vi "Lab Panel V5.28.vi"() -> ()   [LabVIEW 2013] (continued)
                            n1774 = local write "run lab05-2"(w3318) -> ()
                            n1775 = local write "DISP LAB05-2"(w3321) -> ()
                          }
                          frame #1 {
                            n1776 = TDMS Close(11:w3322) -> (0:w3323:errorcluster)  [unwired: 1 in, 1 out]
                            n1777 = local write "data file error"(w3323) -> ()
                          }
                          frame #2 {
                            n1778 = stacked-sequence {
                              tunnel: "LAB05-2" -> [w3331 w3337]
                              tunnel: w3328 -> [_ w3336]
                              tunnel: w3327 -> [_ w3335]
                              tunnel: w3326 -> [_ w3334]
                              tunnel: w3325 -> [_ w3333]
                              tunnel: w3324 -> [_ w3332]
                              frame #0 {
                                n1779 = call "sub vi - defrag tdms v1.vi"("panel id"=w3331) -> ("error out"=w3330:errorcluster)  [unwired: 10 in]
                                n1780 = local write "data file error"(w3330) -> ()
                              }
                              frame #1 {
                                n1781 = Bundle("STATUS"=w3336, "OUT SERVER ADDRESS"=w3335, "FROM ACCOUNT"=w3334, "Mail Test File To:"=w3333, "Mail Test Fail"=w3332) -> (w3339:T26)  [unwired: 1 in]
                                n1782 = call "Save data file (pass-fail) v5.vi"("Input Cluster"=w3339, "panel id"=w3337) -> ("network file save error"=w3338:errorcluster)  [unwired: 8 in, 1 out]
                                n1783 = local write "data file error"(w3338) -> ()
                              }
                            }
                          }
                        }
                      }
                    }
                  }
                }
              }
            }
            n1784 = global write "Global display 2.vi" "Mail test file to:"(w2847) -> ()
            n1785 = local read "Network Directory"() -> (w2853:path)
            n1786 = global write "Global 1.vi" "Network Drive"(w2853) -> ()
          }
          frame #8 {
            # "disable functions"
            n1787 = stacked-sequence {
              tunnel: w3349 -> [w3363 _ w3420]
              tunnel: w3348 -> [w3358 _ w3419]
              tunnel: w3347 -> [w3357 _ w3418]
              tunnel: w3346 -> [w3355 _ w3417]
              tunnel: w3345 -> [w3356 _ w3416]
              tunnel: w3344 -> [_ w3380 w3415]
              tunnel: w3343 -> [_ w3381 w3414]
              tunnel: w3342 -> [_ w3382 w3413]
              tunnel: w3341 -> [_ w3383 w3412]
              tunnel: w3340 -> [_ w3384 w3411]
              frame #0 {
                n1788 = Select(t=2, s=w3355, f=0) -> (s? t:f=w3351:i32)
                n1789 = Select(t=2, s=w3357, f=0) -> (s? t:f=w3352:i32)
                n1790 = Select(t=2, s=w3356, f=0) -> (s? t:f=w3350:i32)
                n1791 = Select(t=2, s=w3363, f=0) -> (s? t:f=w3354:i32)
                n1792 = Select(t=2, s=w3358, f=0) -> (s? t:f=w3353:i32)
                n1793 = property on="SELECT LAB02-2" class="RadioBtnsControl (strict)"("DisabledEnum"=w3351) -> ()  [unwired: 2 in, 2 out]
                n1794 = property on="SELECT LAB02-1" class="RadioBtnsControl (strict)"("DisabledEnum"=w3352) -> ()  [unwired: 2 in, 2 out]
                n1795 = property on="SELECT LAB03-1" class="RadioBtnsControl (strict)"("DisabledEnum"=w3350) -> ()  [unwired: 2 in, 2 out]
                n1796 = property on="SELECT LAB01-1" class="RadioBtnsControl (strict)"("DisabledEnum"=w3354) -> ()  [unwired: 2 in, 2 out]
                n1797 = property on="SELECT LAB01-2" class="RadioBtnsControl (strict)"("DisabledEnum"=w3353) -> ()  [unwired: 2 in, 2 out]
                n1798 = Not(x=w3363) -> (.not. x?=w3364:bool)
                n1799 = property on="RESULT LAB01-1" class="Bool (strict)"("Visible"=w3364) -> ()  [unwired: 2 in, 2 out]
                n1800 = Not(x=w3358) -> (.not. x?=w3362:bool)
                n1801 = Not(x=w3357) -> (.not. x?=w3361:bool)
                n1802 = Not(x=w3355) -> (.not. x?=w3360:bool)
                n1803 = property on="RESULT LAB01-2" class="Bool (strict)"("Visible"=w3362) -> ()  [unwired: 2 in, 2 out]
                n1804 = Not(x=w3356) -> (.not. x?=w3359:bool)
                n1805 = property on="RESULT LAB02-1" class="Bool (strict)"("Visible"=w3361) -> ()  [unwired: 2 in, 2 out]
                n1806 = property on="RESULT LAB02-2" class="Bool (strict)"("Visible"=w3360) -> ()  [unwired: 2 in, 2 out]
                n1807 = property on="RESULT LAB03-1" class="Bool (strict)"("Visible"=w3359) -> ()  [unwired: 2 in, 2 out]
                n1808 = property on="SET LAB01-1" class="Clust (strict)"("DisabledEnum"=w3354) -> ()  [unwired: 2 in, 2 out]
                n1809 = property on="SET LAB01-2" class="Clust (strict)"("DisabledEnum"=w3353) -> ()  [unwired: 2 in, 2 out]
                n1810 = property on="SET LAB02-1" class="Clust (strict)"("DisabledEnum"=w3352) -> ()  [unwired: 2 in, 2 out]
                n1811 = property on="SET LAB02-2" class="Clust (strict)"("DisabledEnum"=w3351) -> ()  [unwired: 2 in, 2 out]
                n1812 = property on="SET LAB03-1" class="Clust (strict)"("DisabledEnum"=w3350) -> ()  [unwired: 2 in, 2 out]
                n1813 = property on="O/I  LAB01-1" class="Bool (strict)"("DisabledEnum"=w3354) -> ()  [unwired: 2 in, 2 out]
                n1814 = property on="O/I  LAB01-2" class="Bool (strict)"("DisabledEnum"=w3353) -> ()  [unwired: 2 in, 2 out]
                n1815 = property on="O/I  LAB02-1" class="Bool (strict)"("DisabledEnum"=w3352) -> ()  [unwired: 2 in, 2 out]
                n1816 = property on="O/I  LAB02-2" class="Bool (strict)"("DisabledEnum"=w3351) -> ()  [unwired: 2 in, 2 out]
                n1817 = property on="O/I  LAB03-1" class="Bool (strict)"("DisabledEnum"=w3350) -> ()  [unwired: 2 in, 2 out]
              }
              frame #1 {
                n1818 = Select(t=2, s=w3384, f=0) -> (s? t:f=w3375:i32)
                n1819 = Select(t=2, s=w3383, f=0) -> (s? t:f=w3376:i32)
                n1820 = Select(t=2, s=w3380, f=0) -> (s? t:f=w3379:i32)
                n1821 = Select(t=2, s=w3381, f=0) -> (s? t:f=w3378:i32)
                n1822 = Select(t=2, s=w3382, f=0) -> (s? t:f=w3377:i32)
                n1823 = property on="SELECT LAB05-2" class="RadioBtnsControl (strict)"("DisabledEnum"=w3375) -> ()  [unwired: 2 in, 2 out]
                n1824 = property on="SELECT LAB05-1" class="RadioBtnsControl (strict)"("DisabledEnum"=w3376) -> ()  [unwired: 2 in, 2 out]
                n1825 = property on="SELECT LAB03-2" class="RadioBtnsControl (strict)"("DisabledEnum"=w3379) -> ()  [unwired: 2 in, 2 out]
                n1826 = property on="SELECT LAB04-1" class="RadioBtnsControl (strict)"("DisabledEnum"=w3378) -> ()  [unwired: 2 in, 2 out]
                n1827 = property on="SELECT LAB04-2" class="RadioBtnsControl (strict)"("DisabledEnum"=w3377) -> ()  [unwired: 2 in, 2 out]
                n1828 = property on="SET LAB05-2" class="Clust (strict)"("DisabledEnum"=w3375) -> ()  [unwired: 2 in, 2 out]
                n1829 = property on="SET LAB05-1" class="Clust (strict)"("DisabledEnum"=w3376) -> ()  [unwired: 2 in, 2 out]
                n1830 = property on="SET LAB03-2" class="Clust (strict)"("DisabledEnum"=w3379) -> ()  [unwired: 2 in, 2 out]
                n1831 = property on="SET LAB04-1" class="Clust (strict)"("DisabledEnum"=w3378) -> ()  [unwired: 2 in, 2 out]
                n1832 = property on="SET LAB04-2" class="Clust (strict)"("DisabledEnum"=w3377) -> ()  [unwired: 2 in, 2 out]
                n1833 = property on="O/I  LAB05-2" class="Bool (strict)"("DisabledEnum"=w3375) -> ()  [unwired: 2 in, 2 out]
                n1834 = property on="O/I  LAB05-1" class="Bool (strict)"("DisabledEnum"=w3376) -> ()  [unwired: 2 in, 2 out]
                n1835 = property on="O/I  LAB04-1" class="Bool (strict)"("DisabledEnum"=w3378) -> ()  [unwired: 2 in, 2 out]
                n1836 = property on="O/I  LAB04-2" class="Bool (strict)"("DisabledEnum"=w3377) -> ()  [unwired: 2 in, 2 out]
                n1837 = property on="O/I  LAB03-2" class="Bool (strict)"("DisabledEnum"=w3379) -> ()  [unwired: 2 in, 2 out]
                n1838 = Not(x=w3384) -> (.not. x?=w3385:bool)
                n1839 = Not(x=w3383) -> (.not. x?=w3386:bool)
                n1840 = Not(x=w3382) -> (.not. x?=w3387:bool)
                n1841 = property on="RESULT LAB05-2" class="Bool (strict)"("Visible"=w3385) -> ()  [unwired: 2 in, 2 out]
                n1842 = property on="RESULT LAB05-1" class="Bool (strict)"("Visible"=w3386) -> ()  [unwired: 2 in, 2 out]
                n1843 = Not(x=w3381) -> (.not. x?=w3388:bool)
                n1844 = property on="RESULT LAB04-2" class="Bool (strict)"("Visible"=w3387) -> ()  [unwired: 2 in, 2 out]
                n1845 = Not(x=w3380) -> (.not. x?=w3389:bool)
                n1846 = property on="RESULT LAB04-1" class="Bool (strict)"("Visible"=w3388) -> ()  [unwired: 2 in, 2 out]
                n1847 = property on="RESULT LAB03-2" class="Bool (strict)"("Visible"=w3389) -> ()  [unwired: 2 in, 2 out]
              }
              frame #2 {
                # "disable calibrate if any test running"
                n1848 = Or(x=w3412, y=w3411) -> (x .or. y?=w3405:bool)
                n1849 = Or(x=w3414, y=w3413) -> (x .or. y?=w3407:bool)
                n1850 = Or(x=w3418, y=w3417) -> (x .or. y?=w3409:bool)
                n1851 = Or(x=w3416, y=w3415) -> (x .or. y?=w3408:bool)
                n1852 = Or(x=w3420, y=w3419) -> (x .or. y?=w3410:bool)
                n1853 = Or(x=w3408, y=w3407) -> (x .or. y?=w3406:bool)
                n1854 = Or(x=w3410, y=w3409) -> (x .or. y?=w3404:bool)
                n1855 = Or(x=w3406, y=w3405) -> (x .or. y?=w3403:bool)
                n1856 = Or(x=w3404, y=w3403) -> (x .or. y?=w3400:bool)
                "Any Test Running" <- w3400
                n1857 = case shown="False" w3400 {
                  tunnel: [0 2] -> w3402
                  frame False {
                  }
                  frame True {
                  }
                }
                n1858 = property on="JIG TEST" class="Clust (strict)"("DisabledEnum"=w3402) -> ()  [unwired: 2 in, 2 out]
                n1859 = property on="Network Directory" class="Path"("DisabledEnum"=w3402) -> ()  [unwired: 2 in, 2 out]
                n1860 = property on="MAIL SETTINGS" class="Clust (strict)"("DisabledEnum"=w3402) -> ()  [unwired: 2 in, 2 out]
                n1861 = property on="SET (cal)" class="Bool (strict)"("DisabledEnum"=w3402) -> ()  [unwired: 2 in, 2 out]
                n1862 = property on="ADMIN" class="Bool (strict)"("DisabledEnum"=0) -> ()  [unwired: 2 in, 2 out]
              }
            }
          }
          frame #9 {
            # "drive jigs"
            n1863 = stacked-sequence {
              frame #0 {
                # "jig on"
                n1864 = local read "jig cycle"() -> (w3428:dbl)
                n1865 = property on="JIG TEST" class="Clust (strict)"() -> ("DisabledEnum"=w3425:T16)  [unwired: 2 in, 2 out]
                n1866 = Equal?(x=w3425, y=2) -> (x = y?=w3424:bool)
                n1867 = Equal?(x=w3428, y=0) -> (x = y?=w3426:bool)
                n1868 = And(x=w3426, y=w3424) -> (x .and. y?=w3423:bool)
                n1869 = case shown="True" w3423 {
                  frame False {
                  }
                  frame True {
                    n1870 = local read "run lab01-1"() -> (w3439:bool)
                    n1871 = local read "run lab01-2"() -> (w3438:bool)
                    n1872 = local read "run lab02-1"() -> (w3437:bool)
                    n1873 = local read "run lab02-2"() -> (w3436:bool)
                    n1874 = local read "run lab03-1"() -> (w3435:bool)
                    n1875 = local read "run lab03-2"() -> (w3434:bool)
                    n1876 = local read "run lab04-1"() -> (w3433:bool)
                    n1877 = local read "run lab04-2"() -> (w3432:bool)
                    n1878 = local read "run lab05-1"() -> (w3431:bool)
                    n1879 = local read "run lab05-2"() -> (w3430:bool)
                    n1880 = local write "JIG LAB03-2"(w3434) -> ()
                    n1881 = local write "JIG LAB01-1"(w3439) -> ()
                    n1882 = local write "JIG LAB01-2"(w3438) -> ()
                    n1883 = local write "JIG LAB02-1"(w3437) -> ()
                    n1884 = local write "JIG LAB02-2"(w3436) -> ()
                    n1885 = local write "JIG LAB03-1"(w3435) -> ()
                    n1886 = local write "JIG LAB04-1"(w3433) -> ()
                    n1887 = local write "JIG LAB04-2"(w3432) -> ()
                    n1888 = local write "JIG LAB05-1"(w3431) -> ()
                    n1889 = local write "JIG LAB05-2"(w3430) -> ()
                  }
                }
              }
              frame #1 {
                # "jig off"
                n1890 = local read "jig cycle"() -> (w3446:dbl)
                n1891 = local read "on loops"() -> (w3445:dbl)
                n1892 = property on="JIG TEST" class="Clust (strict)"() -> ("DisabledEnum"=w3444:T16)  [unwired: 2 in, 2 out]
                n1893 = Equal?(x=w3444, y=2) -> (x = y?=w3442:bool)
                n1894 = Equal?(x=w3446, y=w3445) -> (x = y?=w3441:bool)
                n1895 = And(x=w3441, y=w3442) -> (x .and. y?=w3440:bool)
                n1896 = case shown="True" w3440 {
                  frame False {
                  }
                  frame True {
                    w3497 = FALSE
                    w3498 = TRUE
                    w3496 = 2
                    n1897 = local read "SELECT LAB05-2"() -> (w3487:T3)
                    n1898 = local read "SELECT LAB04-2"() -> (w3489:T3)
                    n1899 = local read "SELECT LAB04-1"() -> (w3490:T3)
                    n1900 = local read "SELECT LAB05-1"() -> (w3488:T3)
                    n1901 = local read "SELECT LAB03-2"() -> (w3491:T3)
                    n1902 = local read "SELECT LAB02-1"() -> (w3494:T3)
                    n1903 = local read "SELECT LAB03-1"() -> (w3492:T3)
                    n1904 = local read "SELECT LAB02-2"() -> (w3493:T3)
                    n1905 = local read "SELECT LAB01-2"() -> (w3495:T3)
                    n1906 = local read "run lab05-1"() -> (w3457:bool)
                    n1907 = local read "run lab05-2"() -> (w3456:bool)
                    n1908 = local read "SELECT LAB01-1"() -> (w3499:T3)
                    n1909 = local read "run lab04-2"() -> (w3458:bool)
                    n1910 = local read "run lab04-1"() -> (w3459:bool)
                    n1911 = local read "run lab01-1"() -> (w3475:bool)
                    n1912 = local read "run lab01-2"() -> (w3464:bool)
                    n1913 = local read "run lab03-2"() -> (w3460:bool)
                    n1914 = local read "run lab03-1"() -> (w3461:bool)
                    n1915 = local read "run lab02-1"() -> (w3463:bool)
                    n1916 = local read "run lab02-2"() -> (w3462:bool)
                    n1917 = Equal?(x=w3496, y=w3492) -> (x = y?=w3470:bool)
                    n1918 = Equal?(x=w3496, y=w3491) -> (x = y?=w3469:bool)
                    n1919 = Equal?(x=w3496, y=w3490) -> (x = y?=w3468:bool)
                    n1920 = Equal?(x=w3496, y=w3489) -> (x = y?=w3467:bool)
                    n1921 = Equal?(x=w3496, y=w3488) -> (x = y?=w3466:bool)
                    n1922 = Equal?(x=w3496, y=w3487) -> (x = y?=w3465:bool)
                    n1923 = Equal?(x=w3496, y=w3499) -> (x = y?=w3476:bool)
                    n1924 = Equal?(x=w3496, y=w3494) -> (x = y?=w3472:bool)
                    n1925 = Equal?(x=w3496, y=w3493) -> (x = y?=w3471:bool)
                    n1926 = Equal?(x=w3496, y=w3495) -> (x = y?=w3473:bool)
                    n1927 = And(x=w3467, y=w3458) -> (x .and. y?=w3449:bool)
                    n1928 = And(x=w3470, y=w3461) -> (x .and. y?=w3452:bool)
                    n1929 = And(x=w3468, y=w3459) -> (x .and. y?=w3450:bool)
                    n1930 = And(x=w3465, y=w3456) -> (x .and. y?=w3447:bool)
                    n1931 = And(x=w3471, y=w3462) -> (x .and. y?=w3453:bool)
                    n1932 = And(x=w3469, y=w3460) -> (x .and. y?=w3451:bool)
                    n1933 = And(x=w3466, y=w3457) -> (x .and. y?=w3448:bool)
                    n1934 = And(x=w3473, y=w3464) -> (x .and. y?=w3455:bool)
                    n1935 = And(x=w3476, y=w3475) -> (x .and. y?=w3474:bool)
                    n1936 = And(x=w3472, y=w3463) -> (x .and. y?=w3454:bool)
                    n1937 = Select(t=w3498, s=w3474, f=w3497) -> (s? t:f=w3477:bool)
                    n1938 = Select(t=w3498, s=w3455, f=w3497) -> (s? t:f=w3478:bool)
                    n1939 = Select(t=w3498, s=w3454, f=w3497) -> (s? t:f=w3479:bool)
                    n1940 = Select(t=w3498, s=w3453, f=w3497) -> (s? t:f=w3480:bool)
                    n1941 = Select(t=w3498, s=w3452, f=w3497) -> (s? t:f=w3481:bool)
                    n1942 = Select(t=w3498, s=w3451, f=w3497) -> (s? t:f=w3482:bool)
                    n1943 = Select(t=w3498, s=w3450, f=w3497) -> (s? t:f=w3483:bool)
                    n1944 = Select(t=w3498, s=w3449, f=w3497) -> (s? t:f=w3484:bool)
                    n1945 = Select(t=w3498, s=w3448, f=w3497) -> (s? t:f=w3485:bool)
                    n1946 = Select(t=w3498, s=w3447, f=w3497) -> (s? t:f=w3486:bool)
                    n1947 = local write "JIG LAB03-2"(w3482) -> ()
                    n1948 = local write "JIG LAB02-1"(w3479) -> ()
                    n1949 = local write "JIG LAB02-2"(w3480) -> ()
                    n1950 = local write "JIG LAB01-2"(w3478) -> ()
                    n1951 = local write "JIG LAB03-1"(w3481) -> ()
                    n1952 = local write "JIG LAB01-1"(w3477) -> ()
                    n1953 = local write "JIG LAB05-2"(w3486) -> ()
                    n1954 = local write "JIG LAB04-1"(w3483) -> ()
                    n1955 = local write "JIG LAB05-1"(w3485) -> ()
                    n1956 = local write "JIG LAB04-2"(w3484) -> ()
                  }
                }
              }
            }
          }
          frame #10 {
            # "enable  jig test output if no test busy"
            n1957 = property on="JIG TEST" class="Clust (strict)"() -> ("DisabledEnum"=w3502:T16)  [unwired: 2 in, 2 out]
            n1958 = Equal?(x=w3502, y=0) -> (x = y?=w3500:bool)
            n1959 = case shown="True" w3500 {
              frame False {
              }
              frame True {
                n1960 = local read "JIG TEST"() -> (w3513:T10)
                n1961 = Unbundle(w3513) -> ("LAB01-1"=w3512:bool, "LAB01-2"=w3511:bool, "LAB02-1"=w3510:bool, "LAB02-2"=w3509:bool, "LAB03-1"=w3508:bool, "LAB03-2"=w3507:bool, "LAB04-1"=w3506:bool, "LAB04-2"=w3505:bool, "LAB05-1"=w3504:bool, "LAB05-2"=w3503:bool)
                n1962 = local write "JIG LAB05-1"(w3504) -> ()
                n1963 = local write "JIG LAB05-2"(w3503) -> ()
                n1964 = local write "JIG LAB04-1"(w3506) -> ()
                n1965 = local write "JIG LAB04-2"(w3505) -> ()
                n1966 = local write "JIG LAB03-2"(w3507) -> ()
                n1967 = local write "JIG LAB01-1"(w3512) -> ()
                n1968 = local write "JIG LAB02-1"(w3510) -> ()
                n1969 = local write "JIG LAB03-1"(w3508) -> ()
                n1970 = local write "JIG LAB01-2"(w3511) -> ()
                n1971 = local write "JIG LAB02-2"(w3509) -> ()
              }
            }
          }
          frame #11 {
            w3514 = FALSE
            # "Drive digital output and reset USB and temperature network if required."
            n1972 = global read "Global display 3.vi" "cycle O/F"() -> (w3523:bool)
            n1973 = local read "O/I  LAB05-2"() -> (w3516:bool)
            n1974 = local read "O/I  LAB05-1"() -> (w3518:bool)
            n1975 = local read "JIG LAB05-2"() -> (w3515:bool)
            n1976 = local read "O/I  LAB04-2"() -> (w3520:bool)
            n1977 = local read "JIG LAB05-1"() -> (w3517:bool)
            n1978 = local read "JIG LAB04-2"() -> (w3519:bool)
            n1979 = local read "O/I  LAB03-1"() -> (w3534:bool)
            n1980 = local read "O/I  LAB04-1"() -> (w3530:bool)
            n1981 = local read "O/I  LAB02-1"() -> (w3538:bool)
            n1982 = local read "O/I  LAB02-2"() -> (w3536:bool)
            n1983 = local read "O/I  LAB03-2"() -> (w3532:bool)
            n1984 = local read "JIG LAB04-1"() -> (w3529:bool)
            n1985 = local read "JIG LAB03-2"() -> (w3531:bool)
            n1986 = local read "O/I  LAB01-2"() -> (w3540:bool)
            n1987 = local read "JIG LAB02-1"() -> (w3537:bool)
            n1988 = local read "JIG LAB02-2"() -> (w3535:bool)
            n1989 = local read "JIG LAB03-1"() -> (w3533:bool)
            n1990 = local read "O/I  LAB01-1"() -> (w3542:bool)
            n1991 = local read "JIG LAB01-2"() -> (w3539:bool)
            n1992 = local read "JIG LAB01-1"() -> (w3541:bool)
            n1993 = case shown="False" w3523 {
              tunnel: [w3655 FALSE] -> w3522
              frame False {
                n1994 = local read "Analog error"() -> (w3657:bool)
                n1995 = local read "Reset Measuring"() -> (w3656:bool)
                n1996 = Or(x=w3656, y=w3657) -> (x .or. y?=w3655:bool)
              }
              frame True {
              }
            }
            n1997 = Build Array(w3535, w3534, w3533, w3532, w3531, w3530, w3529) -> (w3527:bool[])
            "USB OUT 1" <- w3527
            n1998 = Build Array(w3542, w3541, w3540, w3539, w3538, w3537, w3536) -> (w3528:bool[])
            "USB OUT 0" <- w3528
            n1999 = Build Array(w3520, w3519, w3518, w3517, w3516, w3515, w3514, w3514) -> (w3526:bool[])
            "USB OUT 2" <- w3526
            n2000 = Not(x=w3523) -> (.not. x?=w3524:bool)
            n2001 = local read "Simulate"() -> (w3525:bool)
            n2002 = And(x=w3524, y=w3522) -> (x .and. y?=w3521:bool)
            n2003 = stacked-sequence {
              tunnel: w3528 -> [w3546 w3552]
              tunnel: w3527 -> [w3545 w3551]
              tunnel: w3526 -> [w3544 w3550]
              tunnel: w3525 -> [w3543 w3553]
              tunnel: w3521 -> [_ w3554]
              frame #0 {
                # "drive outputs for normal use"
                n2004 = case shown="False" w3543 {
                  tunnel: w3546 -> [w3549 _]
                  tunnel: w3545 -> [w3548 _]
                  tunnel: w3544 -> [w3547 _]
                  frame False {
                    n2005 = call "sub vi - Drive Relays All v6.vi"("Array #2"=w3547, "Array #1"=w3548, "Array #0"=w3549) -> ()  [unwired: 8 in, 1 out]
                  }
                  frame True {
                  }
                }
              }
              frame #1 {
                # "USB  reset routine"
                n2006 = case shown="True" w3554 {
                  tunnel: w3553 -> [_ w3558]
                  tunnel: w3552 -> [_ w3557]
                  tunnel: w3551 -> [_ w3556]
                  tunnel: w3550 -> [_ w3555]
                  frame False {
                  }
                  frame True {
                    n2007 = stacked-sequence {
                      seq-local: [w3560 _ _ _ _] -> [_ w3566 _ _ _]
                      tunnel: w3558 -> [_ w3570 _ _ _]
                      tunnel: w3557 -> [_ w3569 _ _ _]
                      tunnel: w3556 -> [_ w3568 _ _ _]
                      tunnel: w3555 -> [_ w3567 _ _ _]
                      frame #0 {
                        n2008 = case shown="False" "Auto Reset" {
                          tunnel: [w3563 FALSE] -> w3561
                          frame False {
                            n2009 = Two Button Dialog(message="System reset") -> (T button?=w3563:bool)  [unwired: 2 in]
                          }
                          frame True {
                          }
                        }
                        n2010 = disable-structure shown="Disabled" {
                          frame Disabled {
                            n2011 = local write "Tab Control 2"(5) -> ()
                          }
                          frame Enabled {
                          }
                        }
                        n2012 = Or(x="Auto Reset", y=w3561) -> (x .or. y?=w3560:bool)
                      }
                      frame #1 {
                        n2013 = case shown="True" w3566 {
                          tunnel: w3570 -> [_ w3576]
                          tunnel: w3569 -> [_ w3575]
                          tunnel: w3568 -> [_ w3574]
                          tunnel: w3567 -> [_ w3573]
                          frame False {
                          }
                          frame True {
                            n2014 = stacked-sequence {
                              tunnel: w3576 -> [_ w3594 _]
                              tunnel: bool[] [] -> [w3579 w3593 w3612]
                              tunnel: w3575 -> [_ _ w3611]
                              tunnel: w3574 -> [w3578 _ w3610]
                              tunnel: w3573 -> [w3577 _ w3609]
                              tunnel: 5000 -> [w3580 _ w3608]
                              frame #0 {
                                # "switch off test stations for system reset"
                                n2015 = stacked-sequence {
                                tunnel: w3580 -> [w3584 w3588 w3590]
                                tunnel: w3579 -> [w3583 w3587 w3591]
                                tunnel: w3578 -> [w3582 _ _]
                                tunnel: w3577 -> [w3581 w3586 _]
                                frame #0 {
                                # "drive 1st 7 inputs"
                                n2016 = call "sub vi - Drive Relays All v6.vi"("Array #2"=w3581, "Array #1"=w3582, "Array #0"=w3583) -> ()  [unwired: 8 in, 1 out]
                                n2017 = call "Message Display V1.vi"("Message"="Delay off LAB 01-1 to 02-1", "Delay mS"=w3584) -> ()  [unwired: 10 in]
                                }
                                frame #1 {
                                # "drive 2nd 7 inputs"
                                n2018 = call "sub vi - Drive Relays All v6.vi"("Array #2"=w3586, "Array #1"=w3587, "Array #0"=w3587) -> ()  [unwired: 8 in, 1 out]
                                n2019 = call "Message Display V1.vi"("Message"="Delay off LAB 02-2 to 04-1", "Delay mS"=w3588) -> ()  [unwired: 10 in]
                                }
                                frame #2 {
                                # "drive 3rd 7 inputs"
                                n2020 = call "sub vi - Drive Relays All v6.vi"("Array #2"=w3591, "Array #1"=w3591, "Array #0"=w3591) -> ()  [unwired: 8 in, 1 out]
                                n2021 = call "Message Display V1.vi"("Message"="Delay off LAB 04-2 to 05-2", "Delay mS"=w3590) -> ()  [unwired: 10 in]
                                }
                                }
                              }
                              frame #1 {
                                # "reset all usb modules"
                                n2022 = stacked-sequence {
                                tunnel: w3594 -> [_ w3599]
                                tunnel: w3593 -> [w3597 _]
                                frame #0 {
                                n2023 = local write "AI Task"(FALSE) -> ()
                                n2024 = call "sub vi - Drive Relays All v6.vi"("Array #2"=bool[] [FALSE, FALSE, FALSE, FALSE, FALSE, FALSE, TRUE, FALSE], "Array #1"=w3597, "Array #0"=w3597) -> ()  [unwired: 8 in, 1 out]
                                }
                                frame #1 {
                                n2025 = call "Reset Meas v 5.vi"("simulate"=w3599) -> ("Reset Error"=w3598:bool)  [unwired: 10 in]
                                n2026 = case shown="False" w3598 {
                                frame False {
                                n2027 = local read "RATE (Hz)"() -> (w3603:dbl)
                                n2028 = local read "SAMPLES"() -> (w3602:dbl)
                                n2029 = call "sub vi - AI USB4704 (3)  Create Task v4.vi"("Rate Hz"=w3603, "Samples"=w3602) -> ("TASK USB 0"=w3606:i32, "TASK USB 1"=w3605:i32, "TASK USB 2"=w3604:i32, "AI Task Er"=w3600:bool)  [unwired: 9 in, 1 out]
                                n2030 = local write "AI Task"(TRUE) -> ()
                                n2031 = local write "Reset Error"(w3600) -> ()
                                n2032 = local write "AI Task2"(w3604) -> ()
                                n2033 = local write "AI Task1"(w3605) -> ()
                                n2034 = local write "AI Task0"(w3606) -> ()
                                }
                                frame True {
                                "Reset Error" <- TRUE
                                }
                                }
                                }
                                }
                              }
                              frame #2 {
                                # "switch test stations back on after reset"
                                n2035 = stacked-sequence {
                                tunnel: w3612 -> [w3616 w3619 _]
                                tunnel: w3611 -> [w3615 w3621 w3626]
                                tunnel: w3608 -> [w3614 w3617 w3623]
                                tunnel: w3610 -> [_ w3620 w3625]
                                tunnel: w3609 -> [_ _ w3622]
                                frame #0 {
                                # "drive 1st 7 inputs"
                                n2036 = call "sub vi - Drive Relays All v6.vi"("Array #2"=w3616, "Array #1"=w3616, "Array #0"=w3615) -> ()  [unwired: 8 in, 1 out]
                                n2037 = call "Message Display V1.vi"("Message"="Delay on LAB 01-1 to 02-1", "Delay mS"=w3614) -> ()  [unwired: 10 in]
                                }
                                frame #1 {
                                # "drive 1st & 2nd outputs"
                                n2038 = call "sub vi - Drive Relays All v6.vi"("Array #2"=w3619, "Array #1"=w3620, "Array #0"=w3621) -> ()  [unwired: 8 in, 1 out]
                                n2039 = call "Message Display V1.vi"("Message"="Delay on LAB 02-2 to 04-1", "Delay mS"=w3617) -> ()  [unwired: 10 in]
                                }
                                frame #2 {
                                n2040 = call "sub vi - Drive Relays All v6.vi"("Array #2"=w3622, "Array #1"=w3625, "Array #0"=w3626) -> ()  [unwired: 8 in, 1 out]
                                n2041 = call "Message Display V1.vi"("Message"="Delay on LAB 04-2 to 05-2", "Delay mS"=w3623) -> ()  [unwired: 10 in]
                                }
                                }
                              }
                            }
                          }
                        }
                      }
                      frame #2 {
                        w3627 = 0
                        w3628 = FALSE
                        # "set all back to zero"
                        n2042 = local read "Total USB resets"() -> (w3630:dbl)
                        n2043 = local read "Resets Done"() -> (w3632:dbl)
                        n2044 = local write "Reset Measuring"(w3628) -> ()
                        n2045 = local write "Analog error"(w3628) -> ()
                        n2046 = local write "Er USB#2"(w3627) -> ()
                        n2047 = local write "Er USB#0"(w3627) -> ()
                        n2048 = local write "Er USB#1"(w3627) -> ()
                        n2049 = local write "Error USB #0"(w3628) -> ()
                        n2050 = local write "Error USB #1"(w3628) -> ()
                        n2051 = local write "Error USB #2"(w3628) -> ()
                        n2052 = Increment(x=w3630) -> (x+1=w3629:dbl)
                        n2053 = Increment(x=w3632) -> (x+1=→"Resets Done":dbl)
                        n2054 = local write "Total USB resets"(w3629) -> ()
                      }
                      frame #3 {
                        # "save reset value"
                        n2055 = String To Path(string="c:\\crabtree\\Set Up\\") -> (path=w3642:path)
                        n2056 = Build Path(base path=w3642, name or relative path="USB resets.bin") -> (appended path=w3635:path)
                        n2057 = Create Folder(path (use dialog)=w3642) -> (error out=w3634:errorcluster)  [unwired: 2 in, 2 out]
                        n2058 = local read "Total USB resets"() -> (w3633:dbl)
                        n2059 = call <vilib>:"Clear Errors.vi"("error in (no error)"=w3634) -> ()  [unwired: 6 in, 1 out]
                        n2060 = Open/Create/Replace File(file path (use dialog)=w3635, operation (0:open)=T17."replace or create") -> (refnum out=w3640:refnum<file>, error out=w3639:errorcluster)  [unwired: 4 in, 1 out]
                        n2061 = Write to Binary File(file (use dialog)=w3640, data=w3633, error in=w3639) -> (refnum out=w3638:refnum<file>, error out=w3637:errorcluster)  [unwired: 3 in, 1 out]
                        n2062 = Close File(refnum=w3638, error in=w3637) -> (error out=w3636:errorcluster)  [unwired: 1 out]
                        n2063 = local write "data file error"(w3636) -> ()
                      }
                      frame #4 {
                        # "mail reset value"
                        n2064 = local read "MAIL SETTINGS"() -> (w3648:T7)
                        n2065 = local read "Total USB resets"() -> (w3652:dbl)
                        n2066 = Unbundle(w3648) -> ("OUT SERVER ADDRESS"=w3654:string, "FROM ACCOUNT"=w3653:string)  [unwired: 5 out]
                        n2067 = Number To Decimal String(number=w3652) -> (decimal integer string=w3650:string)  [unwired: 1 in]
                        n2068 = Concatenate Strings("Total USB resets: ", w3650) -> (w3649:string)
                        n2069 = call "sub vi - send mail v5.vi"("TO:"="francois@ffg.net", "subject"=w3649, "from"=w3653, "out going server"=w3654) -> ("error out"=w3647:errorcluster)  [unwired: 11 in]
                        n2070 = Bundle(cluster=w3648, "mail error"=w3647) -> (w3646:T7)  [unwired: 6 in]
                        n2071 = local write "MAIL SETTINGS"(w3646) -> ()
                      }
                    }
                  }
                }
              }
            }
          }
          frame #12 {
            # "if all test panels are off stop analog read"
            n2072 = local read "O/I  LAB03-1"() -> (w3680:bool)
            n2073 = local read "O/I  LAB03-2"() -> (w3679:bool)
            n2074 = local read "O/I  LAB04-1"() -> (w3678:bool)
            n2075 = local read "O/I  LAB04-2"() -> (w3677:bool)
            n2076 = local read "O/I  LAB05-1"() -> (w3676:bool)
            n2077 = local read "O/I  LAB05-2"() -> (w3675:bool)
            n2078 = local read "O/I  LAB02-2"() -> (w3681:bool)
            n2079 = local read "O/I  LAB02-1"() -> (w3682:bool)
            n2080 = local read "O/I  LAB01-2"() -> (w3683:bool)
            n2081 = local read "O/I  LAB01-1"() -> (w3684:bool)
            n2082 = Or(x=w3676, y=w3675) -> (x .or. y?=w3673:bool)
            n2083 = Or(x=w3678, y=w3677) -> (x .or. y?=w3674:bool)
            n2084 = Or(x=w3682, y=w3681) -> (x .or. y?=w3672:bool)
            n2085 = Or(x=w3680, y=w3679) -> (x .or. y?=w3670:bool)
            n2086 = Or(x=w3684, y=w3683) -> (x .or. y?=w3671:bool)
            n2087 = Or(x=w3674, y=w3673) -> (x .or. y?=w3667:bool)
            n2088 = Or(x=w3671, y=w3672) -> (x .or. y?=w3669:bool)
            n2089 = Or(x=w3669, y=w3670) -> (x .or. y?=w3668:bool)
            n2090 = local read "Any Test Running"() -> (w3666:bool)
            n2091 = Or(x=w3668, y=w3667) -> (x .or. y?=w3665:bool)
            n2092 = local read "AI Task"() -> (w3661:bool)
            n2093 = Or(x=w3665, y=w3666) -> (x .or. y?=w3660:bool)
            n2094 = Not(x=w3660) -> (.not. x?=w3664:bool)
            n2095 = Not(x=w3661) -> (.not. x?=w3662:bool)
            n2096 = And(x=w3664, y=w3661) -> (x .and. y?=w3663:bool)
            n2097 = And(x=w3660, y=w3662) -> (x .and. y?=w3659:bool)
            n2098 = case shown="True" w3663 {
              frame False {
              }
              frame True {
                # "close task if no test"
                n2099 = local write "AI Task"(FALSE) -> ()
                n2100 = call "sub vi - AI USB4704 (3)  Close Task v2.vi"() -> ()  [unwired: 16 in]
              }
            }
            n2101 = case shown="True" w3659 {
              frame False {
              }
              frame True {
                # "create task for test"
                n2102 = local read "SAMPLES"() -> (w3686:dbl)
                n2103 = local read "RATE (Hz)"() -> (w3685:dbl)
                n2104 = call "sub vi - AI USB4704 (3)  Create Task v4.vi"("Rate Hz"=w3685, "Samples"=w3686) -> ("TASK USB 0"=w3687:i32, "TASK USB 1"=w3688:i32, "TASK USB 2"=w3689:i32)  [unwired: 9 in, 2 out]
                n2105 = local write "AI Task0"(w3687) -> ()
                n2106 = local write "AI Task1"(w3688) -> ()
                n2107 = local write "AI Task2"(w3689) -> ()
                n2108 = local write "AI Task"(TRUE) -> ()
              }
            }
          }
          frame #13 {
            # "get all analog values from USB devices"
            n2109 = local read "on loops"() -> (w3699:dbl)
            n2110 = local read "jig cycle"() -> (w3696:dbl)
            n2111 = Add(x=w3699, y=3) -> (x+y=w3697:dbl)
            n2112 = Equal?(x=w3696, y=3) -> (x = y?=w3694:bool)
            n2113 = Equal?(x=w3696, y=w3697) -> (x = y?=w3695:bool)
            n2114 = Or(x=w3694, y=w3695) -> (x .or. y?=w3693:bool)
            n2115 = global write "Global display 3.vi" "cycle O/F"(w3694) -> ()
            n2116 = case shown="True" w3693 {
              tunnel: w3694 -> [_ w3705]
              tunnel: w3692 -> [_ w3702]
              frame False {
              }
              frame True {
                n2117 = local read "Simulate"() -> (w3708:bool)
                n2118 = case shown="False" w3708 {
                  tunnel: [w3724 dynamicdata[] [] ("array GRAPH")] -> w3714
                  tunnel: [w3723 w3749] -> w3713
                  tunnel: [w3722 w3749] -> w3712
                  tunnel: [w3721 w3749] -> w3711
                  tunnel: [w3720 w3749] -> w3710
                  tunnel: [w3719 w3749] -> w3709
                  tunnel: w3705 -> [_ w3753]
                  tunnel: [w3718 "Ambient Volts"] -> w3704
                  tunnel: [w3717 bool[] []] -> w3703
                  tunnel: w3702 -> [w3716 _]
                  tunnel: [w3715 0.3 ("Analog loop time")] -> w3701
                  frame False {
                    # "analog in"
                    n2119 = case shown="True" w3716 {
                      tunnel: [dynamicdata[] [] ("array GRAPH") w3743] -> w3724
                      tunnel: [w3726 w3742] -> w3723
                      tunnel: [w3726 w3741] -> w3722
                      tunnel: [w3726 w3740] -> w3721
                      tunnel: [w3726 w3739] -> w3720
                      tunnel: [w3726 w3738] -> w3719
                      tunnel: [3 w3737] -> w3718
                      tunnel: [bool[] [] w3736] -> w3717
                      tunnel: [0.0 w3732] -> w3715
                      frame False {
                        w3727 = 0.0
                        # "no test"
                        n2120 = Bundle(w3727, w3727, w3727, w3727, w3727, w3727) -> (w3726:cluster{dbl, dbl, dbl, dbl, dbl, dbl})  [unwired: 1 in]
                      }
                      frame True {
                        # "test on"
                        n2121 = local read "AI data 0"() -> (w3735:waveform(dbl)[])
                        n2122 = local read "AI data 1"() -> (w3734:waveform(dbl)[])
                        n2123 = local read "AI data 2"() -> (w3731:waveform(dbl)[])
                        n2124 = local read "AI Error"() -> (w3733:errorcluster[])
                        n2125 = call "sub vi - Read Analog All v9.5.vi"("data 0"=w3735, "data 1"=w3734, "data 2"=w3731, "AI Error"=w3733) -> ("array GRAPH"=w3743:dynamicdata[], "LAB01"=w3742:T27, "LAB02"=w3741:T28, "LAB03"=w3740:T29, "LAB04"=w3739:T30, "deg C"=w3737:dbl, "USB Error"=w3736:bool[], "LAB05"=w3738:T31)  [unwired: 4 in]
                        n2126 = local read "AI loop time"() -> (w3732:dbl)
                      }
                    }
                  }
                  frame True {
                    # "simulate"
                    n2127 = local read "ON amps"() -> (w3747:dbl)
                    n2128 = local read "OFF amps"() -> (w3748:dbl)
                    n2129 = local read "VOLTS"() -> (w3751:dbl)
                    n2130 = local read "PF"() -> (w3750:dbl)
                    n2131 = Select(t=w3747, s=w3753, f=w3748) -> (s? t:f=w3752:dbl)
                    n2132 = Bundle("OFF amps"=w3752, "VOLTS"=w3751, "PF"=w3750, "OFF amps"=w3752, "VOLTS"=w3751, "PF"=w3750) -> (w3749:T32)  [unwired: 1 in]
                  }
                }
                n2133 = local read "Simulate"() -> (w3707:bool)
                n2134 = stacked-sequence {
                  seq-local: [w3757 _ _ _ _ _ _ _] -> [_ _ _ _ _ _ _ _]
                  seq-local: [w3756 _ _ _ _ _ _ _] -> [_ _ _ _ _ _ _ _]
                  seq-local: [w3755 _ _ _ _ _ _ _] -> [_ _ _ _ _ _ _ w3950]
                  tunnel: w3714 -> [_ w3808 _ _ _ _ _ _]
                  tunnel: w3713 -> [_ _ w3835 _ _ _ _ _]
                  tunnel: w3712 -> [_ _ _ w3863 _ _ _ _]
                  tunnel: w3711 -> [_ _ _ _ w3891 _ _ _]
                  tunnel: w3710 -> [_ _ _ _ _ w3919 _ _]
                  tunnel: w3709 -> [_ _ _ _ _ _ w3947 _]
                  tunnel: w3707 -> [_ _ w3834 w3862 w3890 w3918 w3946 w3952]
                  tunnel: T14 {"1  (A) cal"=1.0, "1 (V) cal"=1.0, "1 (PF) cal"=1.0, "1 (TL) cal"=1.0, "1 (TN) cal"=1.0, "2 (A) cal"=1.0, "2 (V) cal"=1.0, "2 (PF) cal"=1.0, "2 (TL) cal"=1.0, "2 (TN) cal"=1.0} ("CAL LAB01") -> [_ _ w3833 w3861 w3889 w3917 w3945 _]
                  tunnel: w3704 -> [_ _ _ _ _ _ _ w3951]
                  tunnel: w3703 -> [w3760 _ _ _ _ _ _ _]
                  tunnel: w3701 -> [_ w3787 _ _ _ _ _ _]
                  frame #0 {
                    n2135 = Index Array(array=w3760, index=2) -> (element=w3755:bool)
                    n2136 = Index Array(array=w3760, index=1) -> (element=w3756:bool)
                    n2137 = Index Array(array=w3760, index=0) -> (element=w3757:bool)
                    n2138 = local write "Error USB #2"(w3755) -> ()
                    n2139 = local write "Error USB #0"(w3757) -> ()
                    n2140 = local write "Error USB #1"(w3756) -> ()
                    n2141 = stacked-sequence {
                      tunnel: w3757 -> [w3764 _ _ _]
                      tunnel: w3756 -> [_ w3769 _ _]
                      tunnel: 0 -> [w3763 w3768 w3773 _]
                      tunnel: w3755 -> [_ _ w3774 _]
                      frame #0 {
                        n2142 = case shown="True" w3764 {
                          tunnel: w3763 -> [w3765 _]
                          frame False {
                            n2143 = local write "Er USB#0"(w3765) -> ()
                          }
                          frame True {
                            n2144 = local read "Er USB#0"() -> (w3767:dbl)
                            n2145 = Increment(x=w3767) -> (x+1=→"Er USB#0":dbl)
                          }
                        }
                      }
                      frame #1 {
                        n2146 = case shown="True" w3769 {
                          tunnel: w3768 -> [w3770 _]
                          frame False {
                            n2147 = local write "Er USB#1"(w3770) -> ()
                          }
                          frame True {
                            n2148 = local read "Er USB#1"() -> (w3772:dbl)
                            n2149 = Increment(x=w3772) -> (x+1=→"Er USB#1":dbl)
                          }
                        }
                      }
                      frame #2 {
                        n2150 = case shown="True" w3774 {
                          tunnel: w3773 -> [w3775 _]
                          frame False {
                            n2151 = local write "Er USB#2"(w3775) -> ()
                          }
                          frame True {
                            n2152 = local read "Er USB#2"() -> (w3777:dbl)
                            n2153 = Increment(x=w3777) -> (x+1=→"Er USB#2":dbl)
                          }
                        }
                      }
                      frame #3 {
                        w3783 = 10
                        n2154 = local read "Er USB#2"() -> (w3784:dbl)
                        n2155 = local read "Er USB#0"() -> (w3786:dbl)
                        n2156 = local read "Er USB#1"() -> (w3785:dbl)
                        n2157 = Greater Or Equal?(x=w3786, y=w3783) -> (x >= y?=w3781:bool)
                        n2158 = Greater Or Equal?(x=w3785, y=w3783) -> (x >= y?=w3780:bool)
                        n2159 = Greater Or Equal?(x=w3784, y=w3783) -> (x >= y?=w3779:bool)
                        n2160 = Or(x=w3781, y=w3780) -> (x .or. y?=w3782:bool)
                        n2161 = Or(x=w3782, y=w3779) -> (x .or. y?=→"Analog error":bool)
                      }
                    }
                  }
                  frame #1 {
                    # "display graph data on ADM page"
                    n2162 = local write "AI loop time"(w3787) -> ()
                    n2163 = local write "AI"(TRUE) -> ()
                    n2164 = Index Array(array=w3808, index=6) -> (element=→"LAB04-1 (GRAPH)":dynamicdata)
                    n2165 = Index Array(array=w3808, index=7) -> (element=→"LAB04-2 (GRAPH)":dynamicdata)
                    n2166 = Index Array(array=w3808, index=9) -> (element=→"LAB05-2 (GRAPH)":dynamicdata)
                    n2167 = Index Array(array=w3808, index=8) -> (element=→"LAB05-1 (GRAPH)":dynamicdata)
                    n2168 = Index Array(array=w3808, index=5) -> (element=→"LAB03-2 (GRAPH)":dynamicdata)
                    n2169 = Index Array(array=w3808, index=0) -> (element=→"LAB01-1 (GRAPH)":dynamicdata)
                    n2170 = Index Array(array=w3808, index=1) -> (element=→"LAB01-2 (GRAPH)":dynamicdata)
                    n2171 = Index Array(array=w3808, index=2) -> (element=→"LAB02-1 (GRAPH)":dynamicdata)
                    n2172 = Index Array(array=w3808, index=3) -> (element=→"LAB02-2 (GRAPH)":dynamicdata)
                    n2173 = Index Array(array=w3808, index=4) -> (element=→"LAB03-1 (GRAPH)":dynamicdata)
                  }
                  frame #2 {
                    n2174 = case shown="False" w3834 {
                      tunnel: [w3836 w3837] -> w3832
                      tunnel: w3833 -> [_ w3837]
                      frame False {
                        n2175 = local read "CAL LAB01"() -> (w3836:T14)
                      }
                      frame True {
                      }
                    }
                    n2176 = Unbundle By Name(w3835) -> ("OFF amps"=w3831:dbl, "VOLTS"=w3830:dbl, "PF"=w3829:dbl, "OFF amps"=w3828:dbl, "VOLTS"=w3827:dbl, "PF"=w3826:dbl)
                    n2177 = Unbundle By Name(w3832) -> ("1  (A) cal"=w3825:dbl, "1 (V) cal"=w3824:dbl, "1 (PF) cal"=w3823:dbl, "2 (A) cal"=w3822:dbl, "2 (V) cal"=w3821:dbl, "2 (PF) cal"=w3820:dbl)  [unwired: 4 out]
                    n2178 = Multiply(x=w3831, y=w3825) -> (x*y=w3818:dbl)
                    n2179 = Multiply(x=w3830, y=w3824) -> (x*y=w3817:dbl)
                    n2180 = Multiply(x=w3829, y=w3823) -> (x*y=w3816:dbl)
                    n2181 = Multiply(x=w3828, y=w3822) -> (x*y=w3814:dbl)
                    n2182 = Multiply(x=w3827, y=w3821) -> (x*y=w3813:dbl)
                    n2183 = Multiply(x=w3826, y=w3820) -> (x*y=w3812:dbl)
                    n2184 = local read "SIG LAB01-1"() -> (w3819:T2)
                    n2185 = local read "SIG LAB01-2"() -> (w3815:T2)
                    n2186 = Bundle By Name(cluster=w3819, "AMPS"=w3818, "VOLTS"=w3817, "PF"=w3816) -> (w3811:T2)
                    n2187 = Bundle By Name(cluster=w3815, "AMPS"=w3814, "VOLTS"=w3813, "PF"=w3812) -> (w3810:T2)
                    n2188 = global write "Global display 1.vi" "SIG LAB01-2"(w3810) -> ()
                    n2189 = global write "Global display 1.vi" "SIG LAB01-1"(w3811) -> ()
                    n2190 = local write "SIG LAB01-2"(w3810) -> ()
                    n2191 = local write "SIG LAB01-1"(w3811) -> ()
                  }
                  frame #3 {
                    n2192 = Unbundle By Name(w3863) -> ("OFF amps"=w3859:dbl, "VOLTS"=w3858:dbl, "PF"=w3857:dbl, "OFF amps"=w3856:dbl, "VOLTS"=w3855:dbl, "PF"=w3854:dbl)
                    n2193 = case shown="True" w3862 {
                      tunnel: [w3864 w3865] -> w3860
                      tunnel: w3861 -> [_ w3865]
                      frame False {
                        n2194 = local read "CAL LAB02"() -> (w3864:T15)
                      }
                      frame True {
                      }
                    }
                    n2195 = Unbundle By Name(w3860) -> ("1  (A) cal"=w3853:dbl, "1 (V) cal"=w3852:dbl, "1 (PF) cal"=w3851:dbl, "2 (A) cal"=w3850:dbl, "2 (V) cal"=w3849:dbl, "2 (PF) cal"=w3848:dbl)  [unwired: 4 out]
                    n2196 = Multiply(x=w3859, y=w3853) -> (x*y=w3846:dbl)
                    n2197 = Multiply(x=w3858, y=w3852) -> (x*y=w3845:dbl)
                    n2198 = Multiply(x=w3857, y=w3851) -> (x*y=w3844:dbl)
                    n2199 = Multiply(x=w3856, y=w3850) -> (x*y=w3842:dbl)
                    n2200 = Multiply(x=w3855, y=w3849) -> (x*y=w3841:dbl)
